vi "PWMToHCDIO.vi"(11 "PWM":dbl) -> (3 "Out":dbl)   [LabVIEW 2019]
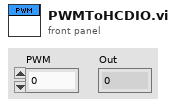
[diagram p1: front panel]
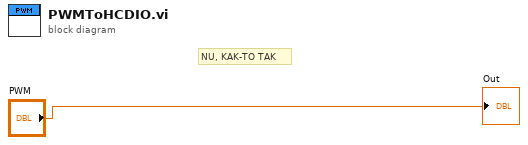
[diagram p0: block diagram]
diagram:
  # "NU, KAK-TO TAK"
  "Out" <- "PWM"
